vi "ServoSmartTurn.vi"(8 "error in":errorcluster, 9 "Turn to (in)":T1=-90 items=["-90°"=-90, "0°"=0, "+90°"=90], 11 "Servo":T2) -> (0 "error out":errorcluster, 3 "Turn to (out)":T1=-90 items=["-90°"=-90, "0°"=0, "+90°"=90])   [LabVIEW 2017]
doc: "Servo turning VI. \nThree turning servos allowed (Left, Front,Right).\nAbsolute angular positions +/-90° and 0°.\n\n1) Configure PWM frequency, conversion from degrees to duty cycle\n2) Assign PWM A channels to servo\n3) (Smart) Open PWM A channel\n4) Move servo, turn to angular positions +90°,0°,-90°\n\nReturns the final position, so that state might be maintained. \n\nExecution type: Preallocated clone reentrant execution\nThe addition of the case structure is necessary to keep the correct status (channel). Otherwise the status of the VI does not correlate to the corresponding servo. Each servo (hardware) demands its own VI (software)."
uses:
  ServoAbsAngleControl.ctl
  ServoEnumControl.ctl
  <vilib>/Utility/error.llb/Error Cluster From Error Code.vi
  <vilib>/myRIO/Common/Instrument Driver Framework/myRIO v1.0/PWM/vis/myRIO v1.0 Write PWM.vi
  <vilib>/myRIO/Instrument Drivers/Onboard IO/PWM/PWM.lvlib
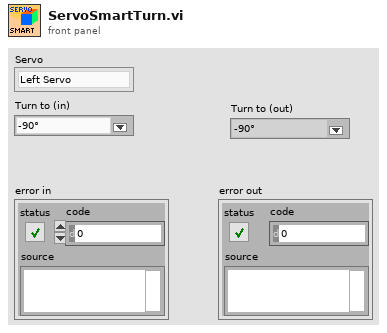
[diagram p1: front panel]
types:
  T1 = typedef "ServoAbsAngleControl.ctl" = i16
  T2 = typedef "ServoEnumControl.ctl" = enum16{"Left Servo", "Front Servo", "Right Servo"}
  T3 = typedef "PWM.lvlib/PWM Reference.ctl" = cluster{"myRIO Reference":T4, "PWM Channels Enum":T8, "PWM Configuration":T9}
  T4 = typedef "myRIO Generic Hardware Reference.ctl" = cluster{"myRIO Model":T5, "myRIO Hardware Reference":T6}
  T5 = typedef "Hardware Version Enum.ctl" = enum16{"Unknown", "myRIO-1900", "myRIO-1950", "roboRIO", "NI ELVIS RIO CM"}
  T6 = typedef "myRIO v1.0 Reference.ctl" = cluster{"Generic FPGA Reference":T7, "Allow multiple opens":bool}
  T7 = typedef "Generic FPGA Reference.ctl" = refnum<k20>
  T8 = typedef "PWM Channels Enum.ctl" = enum16{"Not Connected", "C/PWM0", "C/PWM1", "A/PWM0", "A/PWM1", "A/PWM2", "B/PWM0", "B/PWM1", "B/PWM2", "PWM/PWM0", "PWM/PWM1", "PWM/PWM2", "PWM/PWM3", "PWM/PWM4", "PWM/PWM5", "PWM/PWM6", "PWM/PWM7", "PWM/PWM8", "PWM/PWM9"}
  T9 = typedef "PWM.lvlib/PWM Configuration.ctl" = cluster{"Frequency":dbl, "Duty Cycle":dbl}
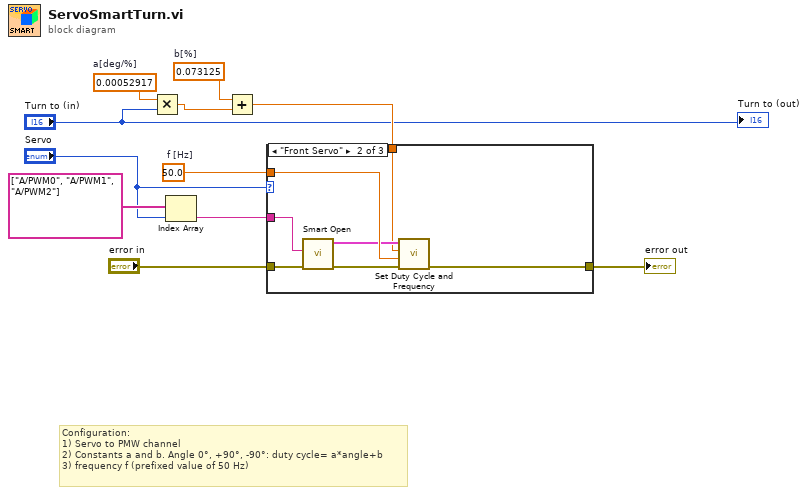
[diagram p0: block diagram]
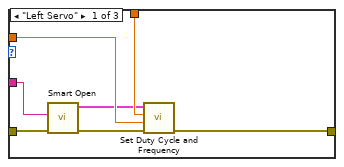
[diagram p2: hidden frame]
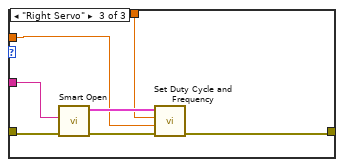
[diagram p3: hidden frame]
diagram:
  w8 = 0.00052917  # a[deg/%]
  w7 = 0.073125  # b[%]
  w11 = 50.0  # f [Hz]
  # "Configuration:\n1) Servo to PMW channel\n2) Constants a and b. Angle 0°, +90°, -90°: duty cycle= a*angle+b\n3) frequency f (prefixed value of 50 Hz)"
  n1 = Multiply(x=w8, y="Turn to (in)") -> (x*y=w6:dbl)
  n2 = Index Array(array=tag[] ["A/PWM0", "A/PWM1", "A/PWM2"], index="Servo") -> (element=w4:tag)
  n3 = Add(x=w7, y=w6) -> (x+y=w3:dbl)
  n4 = case shown="\"Front Servo\"" "Servo" {
    tunnel: w11 -> [w16 w25 w26]
    tunnel: "error in" -> [w14 w24 w29]
    tunnel: [w15 w21 w30] -> w9
    tunnel: w4 -> [w13 w20 w28]
    tunnel: w3 -> [w17 w19 w27]
    frame "Left Servo" {
      n5 = call <vilib>:"Smart Open.vi"("error in (no error)"=w14, "Channel Name"=w13) -> ("error out"=w18:errorcluster, "PWM Ref Out"=w12:T3)  [unwired: 8 in]
      n6 = call <vilib>:"Set Duty Cycle and Frequency.vi"("error in (no error)"=w18, "Frequency [Hz]"=w16, "Duty Cycle"=w17, "PWM Ref In"=w12) -> ("error out"=w15:errorcluster)  [unwired: 5 in, 1 out]
    }
    frame "Front Servo" {
      n7 = call <vilib>:"Smart Open.vi"("error in (no error)"=w24, "Channel Name"=w20) -> ("error out"=w22:errorcluster, "PWM Ref Out"=w23:T3)  [unwired: 8 in]
      n8 = call <vilib>:"Set Duty Cycle and Frequency.vi"("error in (no error)"=w22, "Frequency [Hz]"=w25, "Duty Cycle"=w19, "PWM Ref In"=w23) -> ("error out"=w21:errorcluster)  [unwired: 5 in, 1 out]
    }
    frame "Right Servo" {
      n9 = call <vilib>:"Smart Open.vi"("error in (no error)"=w29, "Channel Name"=w28) -> ("error out"=w32:errorcluster, "PWM Ref Out"=w31:T3)  [unwired: 8 in]
      n10 = call <vilib>:"Set Duty Cycle and Frequency.vi"("error in (no error)"=w32, "Frequency [Hz]"=w26, "Duty Cycle"=w27, "PWM Ref In"=w31) -> ("error out"=w30:errorcluster)  [unwired: 5 in, 1 out]
    }
  }
  "error out" <- w9
  "Turn to (out)" <- "Turn to (in)"
